vi "User Interface.vi"(8 "error in":errorcluster, 11 "User Interface in":refnum<class "User Interface.lvclass">) -> (0 "error out":errorcluster, 3 "User Interface out":refnum<class "User Interface.lvclass">)   [LabVIEW 2020, in "RDMA.lvlib" / "RDMA Transfer Tx User Interface.lvclass"]
uses:
  RDMA Transfer Tx User Interface.lvclass
  DSF Core.lvlibp/Classes/User Interface/User Interface.lvclass
  Configuration/Tx Transfer/RDMA Transfer Tx Configuration.lvclass
  C:/dev/niveristand-data-sharing-framework-custom-device-plugins/Components/DSF Core.lvlibp/Classes/Configuration/Configuration.lvclass
  C:/dev/niveristand-data-sharing-framework-custom-device-plugins/Components/Transceivers/RDMA/Configuration/Tx Transfer/RDMA Transfer Tx Configuration.lvclass
panel:
  in  "Decimation":u16
  in  "Local Port":u16
  in  "Local Address":string
  in  "Destination Address":string
  in  "Destination Port":u16
  # "RDMA Plugin Settings"
  # "* The address fields must be in IP dot notation. \n   Example: 10.0.53.23"
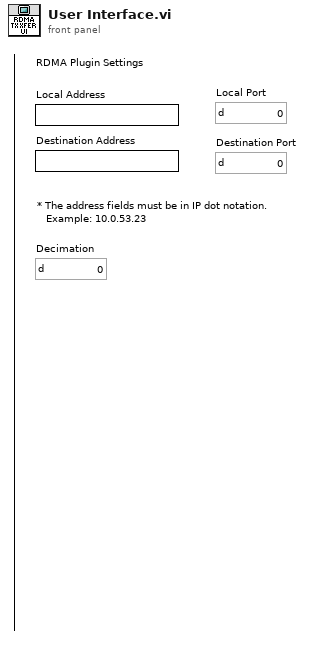
[diagram p1: front panel]
types:
  T1 = typedef "RDMA.lvlib/RDMA Transfer Tx Configuration.lvclass/Tx Transfer Settings.ctl" = cluster{"local address":u32, "local port":u16, "destination address":u32, "destination port":u16, "decimation":u16}
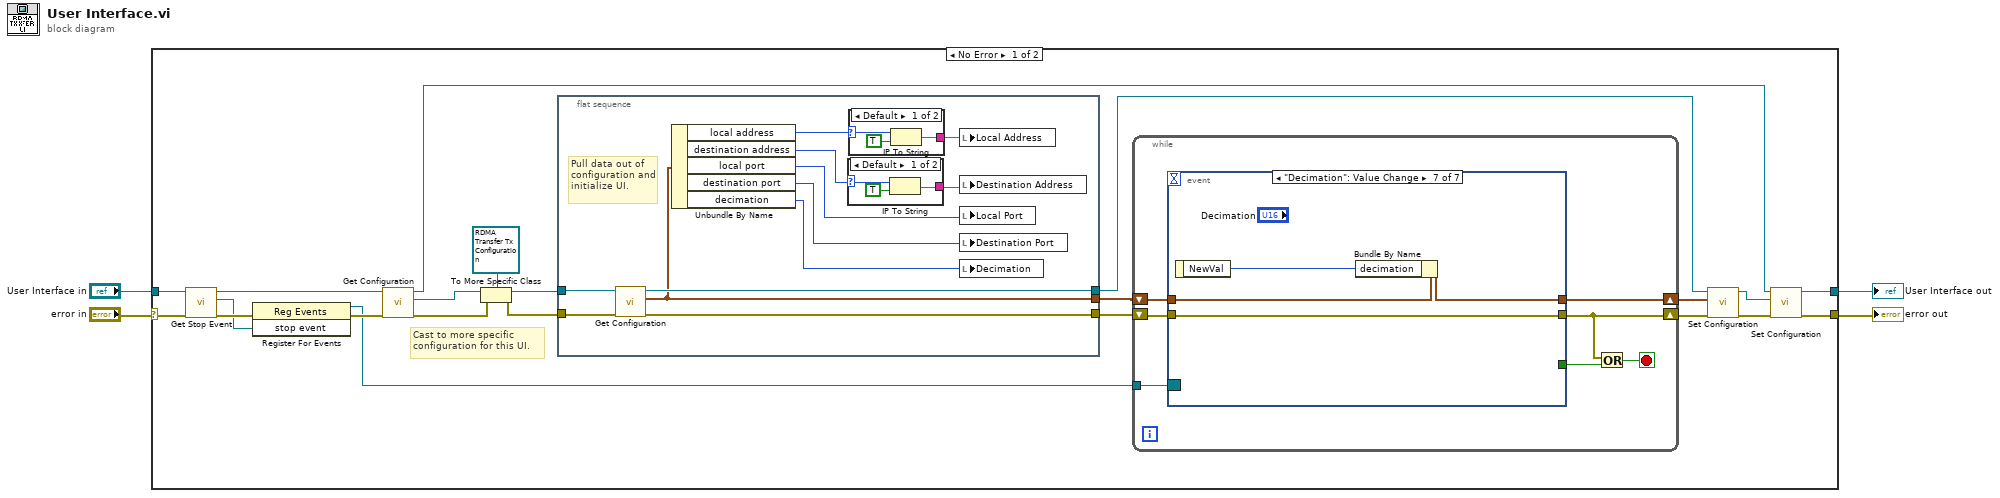
[diagram p0: block diagram]
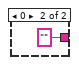
[diagram p2: hidden frame]
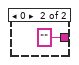
[diagram p3: hidden frame]
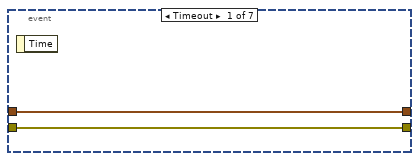
[diagram p4: hidden frame]
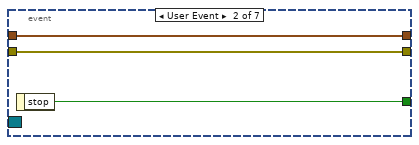
[diagram p5: hidden frame]
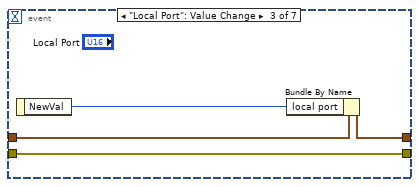
[diagram p6: hidden frame]
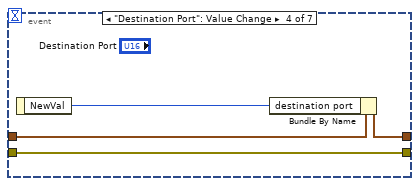
[diagram p7: hidden frame]
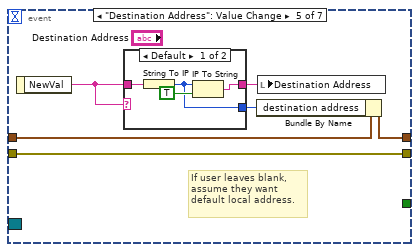
[diagram p8: hidden frame]
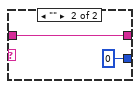
[diagram p9: hidden frame]
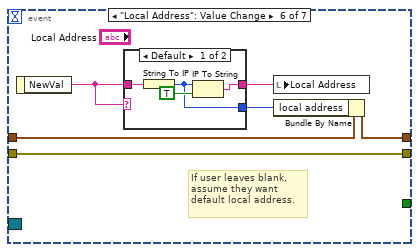
[diagram p10: hidden frame]
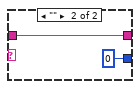
[diagram p11: hidden frame]
diagram:
  n1 = case shown="No Error" "error in" {
    selector: "error in" -> [w26 w96]
    tunnel: [w17 w96] -> w4
    tunnel: "User Interface in" -> [w25 w95]
    tunnel: [w16 w95] -> w1
    frame No Error {
      # "Cast to more specific configuration for this UI."
      n2 = call "Get Stop Event.vi"("error in (no error)"=w26, "User Interface in"=w25) -> ("error out"=w24:errorcluster, "stop event"=w23:refnum<user-event>, "User Interface out"=w22:refnum<class "User Interface.lvclass">)  [unwired: 7 in]
      n3 = register-events(error in=w24, w23) -> (reference out=w20:refnum<event-registration>, error out=w21:errorcluster)  [unwired: 1 in]
      n4 = call "Get Configuration.vi"("error in (no error)"=w21, "User Interface in"=w22) -> ("error out"=w19:errorcluster, "configuration"=w18:refnum<class "Configuration.lvclass">, "User Interface out"=w15:refnum<class "User Interface.lvclass">)  [unwired: 7 in]
      n5 = To More Specific Class(target class=refnum<class "RDMA Transfer Tx Configuration.lvclass"> refnum ("DSF Core.lvlib:UDP Transfer Tx Configuration.lvclass"), reference=w18, error in=w19) -> (specific class reference=w9:refnum<class "RDMA Transfer Tx Configuration.lvclass">, error out=w8:errorcluster)
      n6 = flat-sequence {
        tunnel: [w36] -> w5
        tunnel: w8 -> [w38]
        tunnel: w9 -> [w37]
        tunnel: [w34] -> w7
        tunnel: [w33] -> w6
        frame #0 {
          # "Pull data out of configuration and initialize UI."
          n7 = call "Get Configuration.vi"("error in"=w38, "RDMA Transfer Tx Configuration in"=w37) -> ("error out"=w36:errorcluster, "transfer settings"=w33:T1, "RDMA Transfer Tx Configuration out"=w34:refnum<class "RDMA Transfer Tx Configuration.lvclass">)  [unwired: 7 in]
          n8 = Unbundle By Name(w33) -> ("local address"=w32:u32, "destination address"=w31:u32, "local port"=w29:u16, "destination port"=w28:u16, "decimation"=w27:u16)
          n9 = case shown="Default" w31 {
            selector: w31 -> [w39 _]
            tunnel: [w41 "" ("name")] -> w30
            frame Default {
              n10 = IP To String(1:TRUE ("dot notation? (F)"), 2:w39) -> (0:w41:string)
            }
            frame 0 {
            }
          }
          n11 = case shown="Default" w32 {
            selector: w32 -> [w43 _]
            tunnel: [w45 "" ("name")] -> w35
            frame Default {
              n12 = IP To String(1:TRUE ("dot notation? (F)"), 2:w43) -> (0:w45:string)
            }
            frame 0 {
            }
          }
          n13 = local write "Local Address"(w35) -> ()
          n14 = local write "Destination Address"(w30) -> ()
          n15 = local write "Local Port"(w29) -> ()
          n16 = local write "Destination Port"(w28) -> ()
          n17 = local write "Decimation"(w27) -> ()
        }
      }
      n18 = while {
        tunnel: w20 -> [w50]
        shift-right: [w48] -> w13
        shift-left: w5 -> [w51]
        shift-right: [w47] -> w11
        shift-left: w6 -> [w52]
        stop <- w53 stop-if-true
        n19 = event shown="[6] \"Decimation\": Value Change" {
          selector: w50 -> [_ _ _ _ _ _ _]
          dyn-events: _ -> [_ _ _ _ _ _ _]
          timeout: _ -> [_ _ _ _ _ _ _]
          tunnel: [_ w57 _ _ _ _ _] -> w49
          tunnel: w51 -> [w55 w58 w62 w66 w69 w81 w92]
          tunnel: [w55 w58 w62 w66 w69 w81 w92] -> w48
          tunnel: w52 -> [w54 w56 w61 w65 w70 w82 w94]
          tunnel: [w54 w56 w60 w64 w72 w84 w93] -> w47
          event Timeout {
            n20 = event-data() -> ()  [unwired: 1 in, 1 out]
          }
          event User Event {
            n21 = event-data() -> ("stop"=w57:bool)  [unwired: 1 in]
          }
          event "Local Port": Value Change {
            n22 = event-data() -> ("NewVal"=w59:u16)  [unwired: 1 in]
            n23 = Bundle By Name(cluster=w61, "local port"=w59) -> (w60:T1)
          }
          event "Destination Port": Value Change {
            n24 = event-data() -> ("NewVal"=w63:u16)  [unwired: 1 in]
            n25 = Bundle By Name(cluster=w65, "destination port"=w63) -> (w64:T1)
          }
          event "Destination Address": Value Change {
            # "If user leaves blank, assume they want default local address."
            n26 = event-data() -> ("NewVal"=w67:string)  [unwired: 1 in]
            n27 = case shown="Default" w67 {
              tunnel: [w76 w77] -> w71
              tunnel: w67 -> [w75 w77]
              tunnel: [w73 u32 0] -> w68
              frame Default {
                n28 = String To IP(1:w75) -> (0:w73:u32)
                n29 = IP To String(1:TRUE ("dot notation? (F)"), 2:w73) -> (0:w76:string)
              }
              frame "" {
              }
            }
            n30 = Bundle By Name(cluster=w70, "destination address"=w68) -> (w72:T1)
            n31 = local write "Destination Address"(w71) -> ()
          }
          event "Local Address": Value Change {
            # "If user leaves blank, assume they want default local address."
            n32 = event-data() -> ("NewVal"=w79:string)  [unwired: 1 in]
            n33 = case shown="Default" w79 {
              tunnel: [w88 w89] -> w83
              tunnel: w79 -> [w87 w89]
              tunnel: [w85 u32 0] -> w80
              frame Default {
                n34 = String To IP(1:w87) -> (0:w85:u32)
                n35 = IP To String(1:TRUE ("dot notation? (F)"), 2:w85) -> (0:w88:string)
              }
              frame "" {
              }
            }
            n36 = local write "Local Address"(w83) -> ()
            n37 = Bundle By Name(cluster=w82, "local address"=w80) -> (w84:T1)
          }
          event "Decimation": Value Change {
            n38 = event-data() -> ("NewVal"=w91:u16)  [unwired: 1 in]
            n39 = Bundle By Name(cluster=w94, "decimation"=w91) -> (w93:T1)
          }
        }
        n40 = Or(x=w48, y=w49) -> (x .or. y?=w53:bool)
      }
      n41 = call "Set Configuration.vi"("error in"=w13, "transfer settings"=w11, "RDMA Transfer Tx Configuration in"=w7) -> ("error out"=w12:errorcluster, "RDMA Transfer Tx Configuration out"=w10:refnum<class "RDMA Transfer Tx Configuration.lvclass">)  [unwired: 7 in]
      n42 = call "Set Configuration.vi"("error in (no error)"=w12, "configuration"=w10, "User Interface in"=w15) -> ("error out"=w17:errorcluster, "User Interface out"=w16:refnum<class "User Interface.lvclass">)  [unwired: 7 in]
    }
    frame Error {
    }
  }
  "error out" <- w4
  "User Interface out" <- w1
